vi "Read PlatMods.vi"(8 "error in (no error)":errorcluster, 11 "ListboxDoubleClickMsg in":refnum<class "ListboxDoubleClickMsg.lvclass">) -> (0 "error out":errorcluster, 2 "PlatMods":T1, 3 "ListboxDoubleClickMsg out":refnum<class "ListboxDoubleClickMsg.lvclass">)   [LabVIEW 2020, in "MVA Framework.lvlib" / "ActorEvents.lvlib" / "ListboxDoubleClickMsg.lvclass"]
uses:
  ListboxDoubleClickMsg.lvclass
  ListboxDoubleClickMsg.lvclass/ListboxDoubleClickMsg.ctl
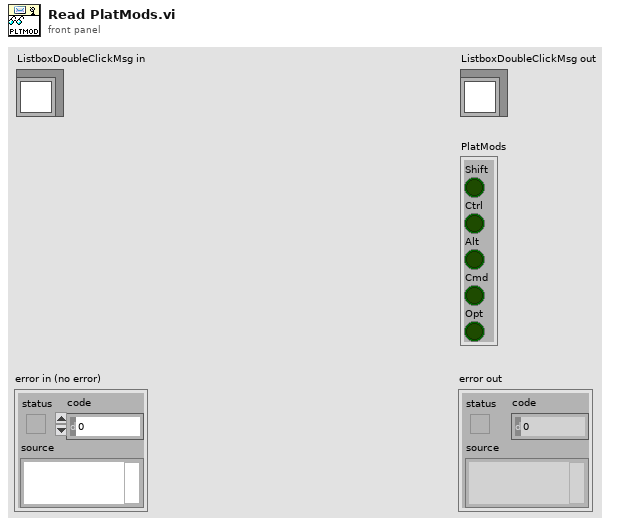
[diagram p1: front panel]
types:
  T1 = cluster{"Shift":bool, "Ctrl":bool, "Alt":bool, "Cmd":bool, "Opt":bool}
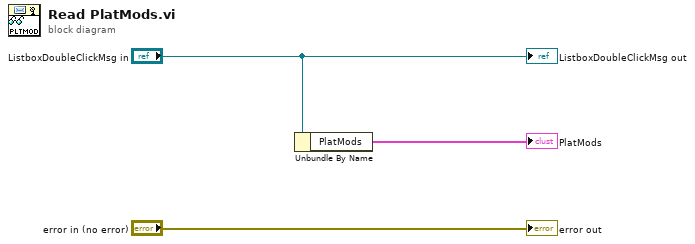
[diagram p0: block diagram]
diagram:
  n1 = Unbundle By Name("ListboxDoubleClickMsg in") -> ("PlatMods"=→"PlatMods":T1)
  "error out" <- "error in (no error)"
  "ListboxDoubleClickMsg out" <- "ListboxDoubleClickMsg in"
